vi "Manual Mode.vi"(8 "error in (no error)":errorcluster, 9 "Test Settings":T1, 10 "Model in":refnum<class "Model.lvclass">, 11 "Wait For User Input State in":refnum<class "Wait For User Input State.lvclass">) -> (0 "error out":errorcluster, 2 "Model out":refnum<class "Model.lvclass">, 3 "Wait For User Input State out":refnum<class "Wait For User Input State.lvclass">)   [LabVIEW 2016, in "Wait For User Input State.lvclass"]
uses:
  Wait For User Input State.lvclass
  Model/Model/Model.lvclass
  Typedefs/TestSettings.ctl
  common_rt_hpilc/HPILCFactory/HPILCFactory.lvclass
  Typedefs/StateTypes.ctl
  Model/Model/Model.lvclass/Model.ctl
  Model/Boot Loader/Boot Loader.lvclass
  Typedefs/HPMT_Typedefs.lvlib
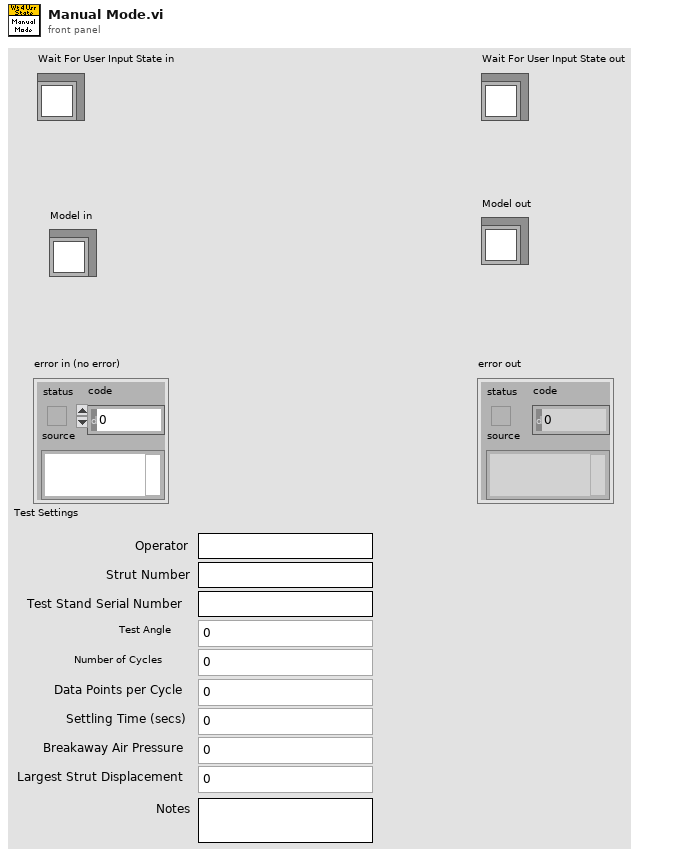
[diagram p1: front panel]
types:
  T1 = typedef "HPMT_Typedefs.lvlib/TestSettings.ctl" = cluster{"Operator":string, "Strut Number":string, "Test Stand Serial Number":string, "Notes":string, "Test Angle":u16, "Number of Cycles":u16, "Data Points per Cycle":u16, "Settling Time (secs)":u16, "Breakaway Air Pressure":u16, "Largest Strut Displacement":dbl}
  T2 = typedef "HPMT_Typedefs.lvlib/StateTypes.ctl" = enum16{"Offline State", "Fault State", "Standby State", "Disabled State", "Enabled State", "Wait For User Input State", "Test Actuator State", "Manual State"}
  T3 = typedef "RTHPILC.lvlib/HPSettings.ctl" = cluster{"ILCSettings":T4, "ID":i16, "ReferencePosition":i32}
  T4 = typedef "RTILC.lvlib/ILCSettings.ctl" = cluster{"Subnet":u8, "Address":u8}
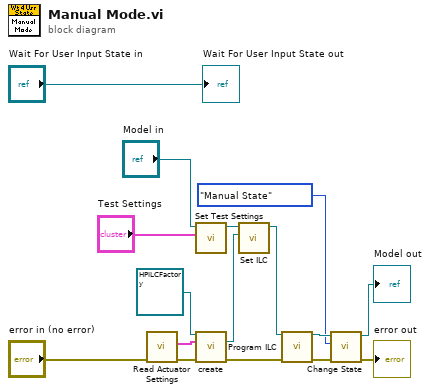
[diagram p0: block diagram]
diagram:
  n1 = call "Read Actuator Settings.vi"("error in (no error)"="error in (no error)") -> ("error out"=w9:errorcluster, "HPSettings"=w12:T3)  [unwired: 8 in, 1 out]
  n2 = call "Set Test Settings.vi"("Test Settings"="Test Settings", "Model in"="Model in") -> ("Model out"=w14:refnum<class "Model.lvclass">)  [unwired: 9 in]
  n3 = call "create.vi"("HPILCFactory in"=refnum<class "HPILCFactory.lvclass"> refnum ("RTHPILC.lvlib:HPILCFactory.lvclass"), "HPSettings"=w12, "error in (no error)"=w9) -> ("HPILC"=w10:refnum<class "HPILC.lvclass">, "error out"=w8:errorcluster)  [unwired: 10 in, 1 out]
  n4 = call "Set ILC.vi"("HPILC"=w10, "Model in"=w14) -> ("Model out"=w7:refnum<class "Model.lvclass">)  [unwired: 9 in]
  n5 = call "Program ILC.vi"("Model in"=w7, "error in (no error)"=w8) -> ("Model out"=w6:refnum<class "Model.lvclass">, "error out"=w5:errorcluster)  [unwired: 12 in]
  n6 = call "Change State.vi"("error in (no error)"=w5, "State Types"=StateTypes."Manual State" ("State:"), "Model in"=w6) -> ("error out"=→"error out":errorcluster, "Model out"=→"Model out":refnum<class "Model.lvclass">)  [unwired: 7 in]
  "Wait For User Input State out" <- "Wait For User Input State in"
